vi "QueueTestReceiver.vi"() -> ()   [LabVIEW 2013]
panel:
  in  "stop 2":bool
  out "RandOut":dbl(graph)
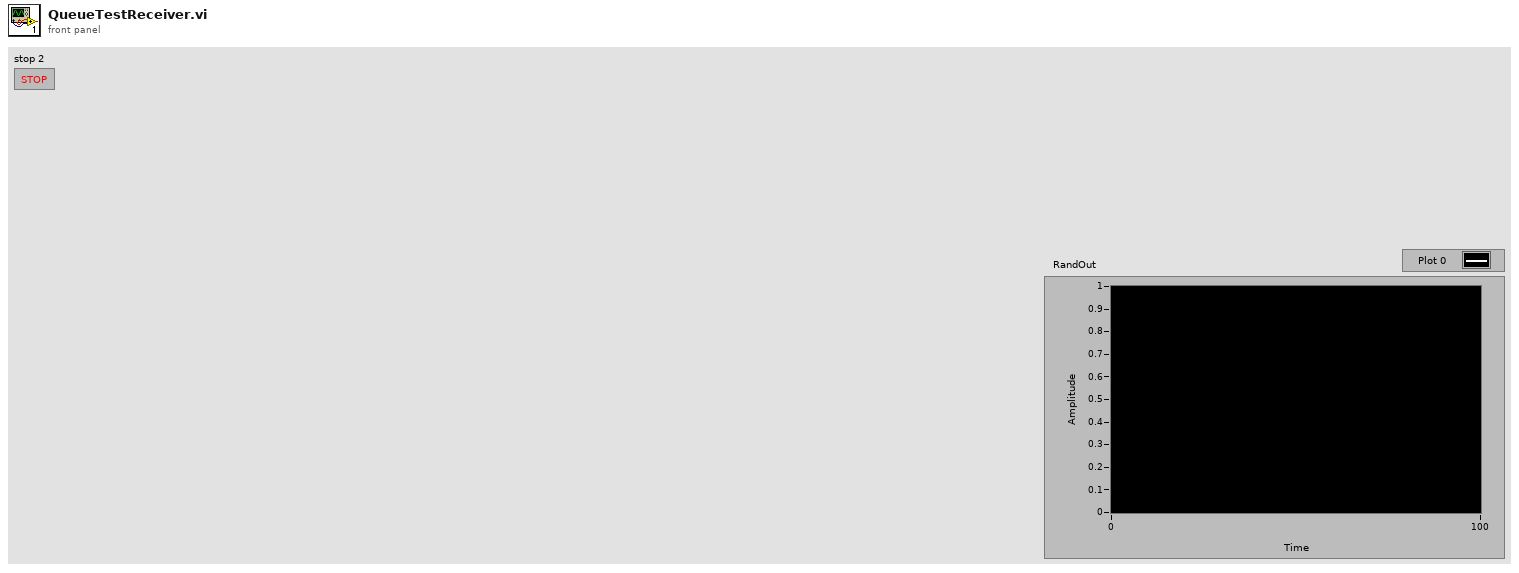
[diagram p1: front panel]
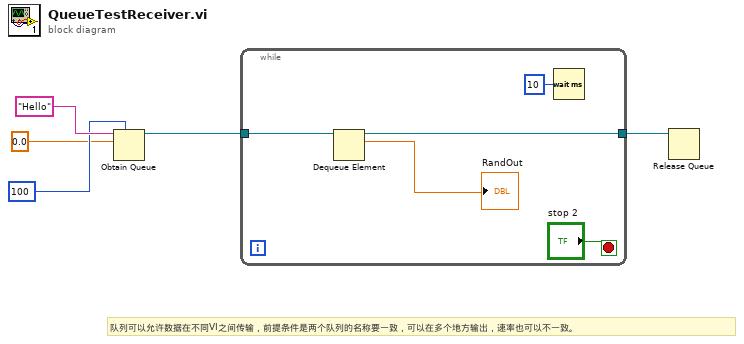
[diagram p0: block diagram]
diagram:
  # "队列可以允许数据在不同VI之间传输，前提条件是两个队列的名称要一致，可以在多个地方输出，速率也可以不一致。"
  n1 = Obtain Queue(max queue size (-1, unlimited)=100, name (unnamed)="Hello", element data type=0.0) -> (queue out=w2:refnum<queue>)  [unwired: 2 in, 2 out]
  n2 = while {
    tunnel: w2 -> [w9]
    tunnel: [w8] -> w1
    stop <- "stop 2" stop-if-true
    n3 = Dequeue Element(queue=w9) -> (queue out=w8:refnum<queue>, element=→"RandOut":dbl)  [unwired: 2 in, 2 out]
    n4 = Wait (ms)(milliseconds to wait=u32 10) -> ()  [unwired: 1 out]
  }
  n5 = Release Queue(queue=w1) -> ()  [unwired: 2 in, 3 out]
